vi "Adjust_PID-Controller.vi"() -> ()   [LabVIEW 2018]
uses:
  <vilib>/robotics/Steering/Wheel/Rotation Direction.ctl
  <vilib>/robotics/Steering/Wheel/Wheel Parameters.ctl
  <vilib>/Studica/Studica Toolkit/Background/Mxp Selection.ctl
  <vilib>/robotics/Steering/Omnidirectional Wheel/NI_Robotics_Omnidirectional Wheel.lvclass
  C:/Program Files (x86)/National Instruments/LabVIEW 2018/vi.lib/robotics/Steering/Wheel/NI_Robotics_Wheel.lvclass
  <vilib>/robotics/Steering/Omnidirectional Wheel/Create Omnidirectional Wheel.vi
  <vilib>/robotics/Steering/Steering Frame/Create User Defined Steering Frame.vi
  <vilib>/robotics/Steering/Steering Frame/Apply Steering Frame Velocity to Motors.vi
  <vilib>/robotics/Steering/Wheel/NI_Robotics_Wheel.lvclass
  <vilib>/robotics/Steering/Steering Frame/NI_Robotics_Steering Frame.lvclass
panel:
  in  "PID gains":T1(array[cluster]) {"proportional gain (Kc)" step=0.01; "integral time (Ti, min)" min=0.0 step=0.0001; "derivative time (Td, min)" step=0.0001}
  out "PID-Output":dbl[](array[numeric])
  out "Actual-SpeedList":dbl[](array[numeric])
  out "Desired Velocity":dbl[](array[numeric])=[-0.0, -0.0, -0.0]
  in  "theta":dbl
  in  "y":dbl
  in  "x":dbl
  in  "Reset Encoders":bool
  out "Tick Count(uSec)":u32=1278617 caption="Tick Count(Ticks)"
  in  "Wheel Index Adjustment (2, 0, 1)":i32[](array[numeric])=[2, 0, 1]
  in  "stop":bool
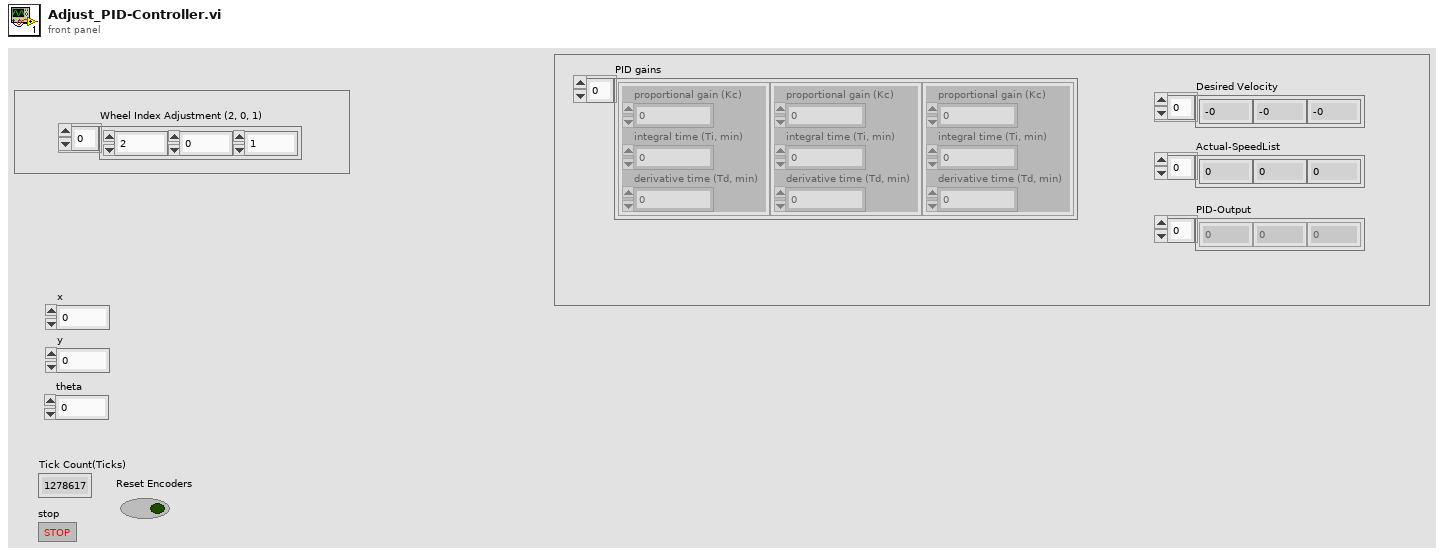
[diagram p1: front panel]
types:
  T1 = cluster{"proportional gain (Kc)":dbl, "integral time (Ti, min)":dbl, "derivative time (Td, min)":dbl}[]
  T2 = typedef "NI_Robotics_Wheel.lvclass/Wheel Parameters.ctl" = cluster{"wheel radius":dbl, "gear ratio":dbl, "forward rotation direction":T3}
  T3 = typedef "NI_Robotics_Wheel.lvclass/Rotation Direction.ctl" = u16
  T4 = typedef "Mxp Selection.ctl" = enum16{"MXP A", "MXP B"}
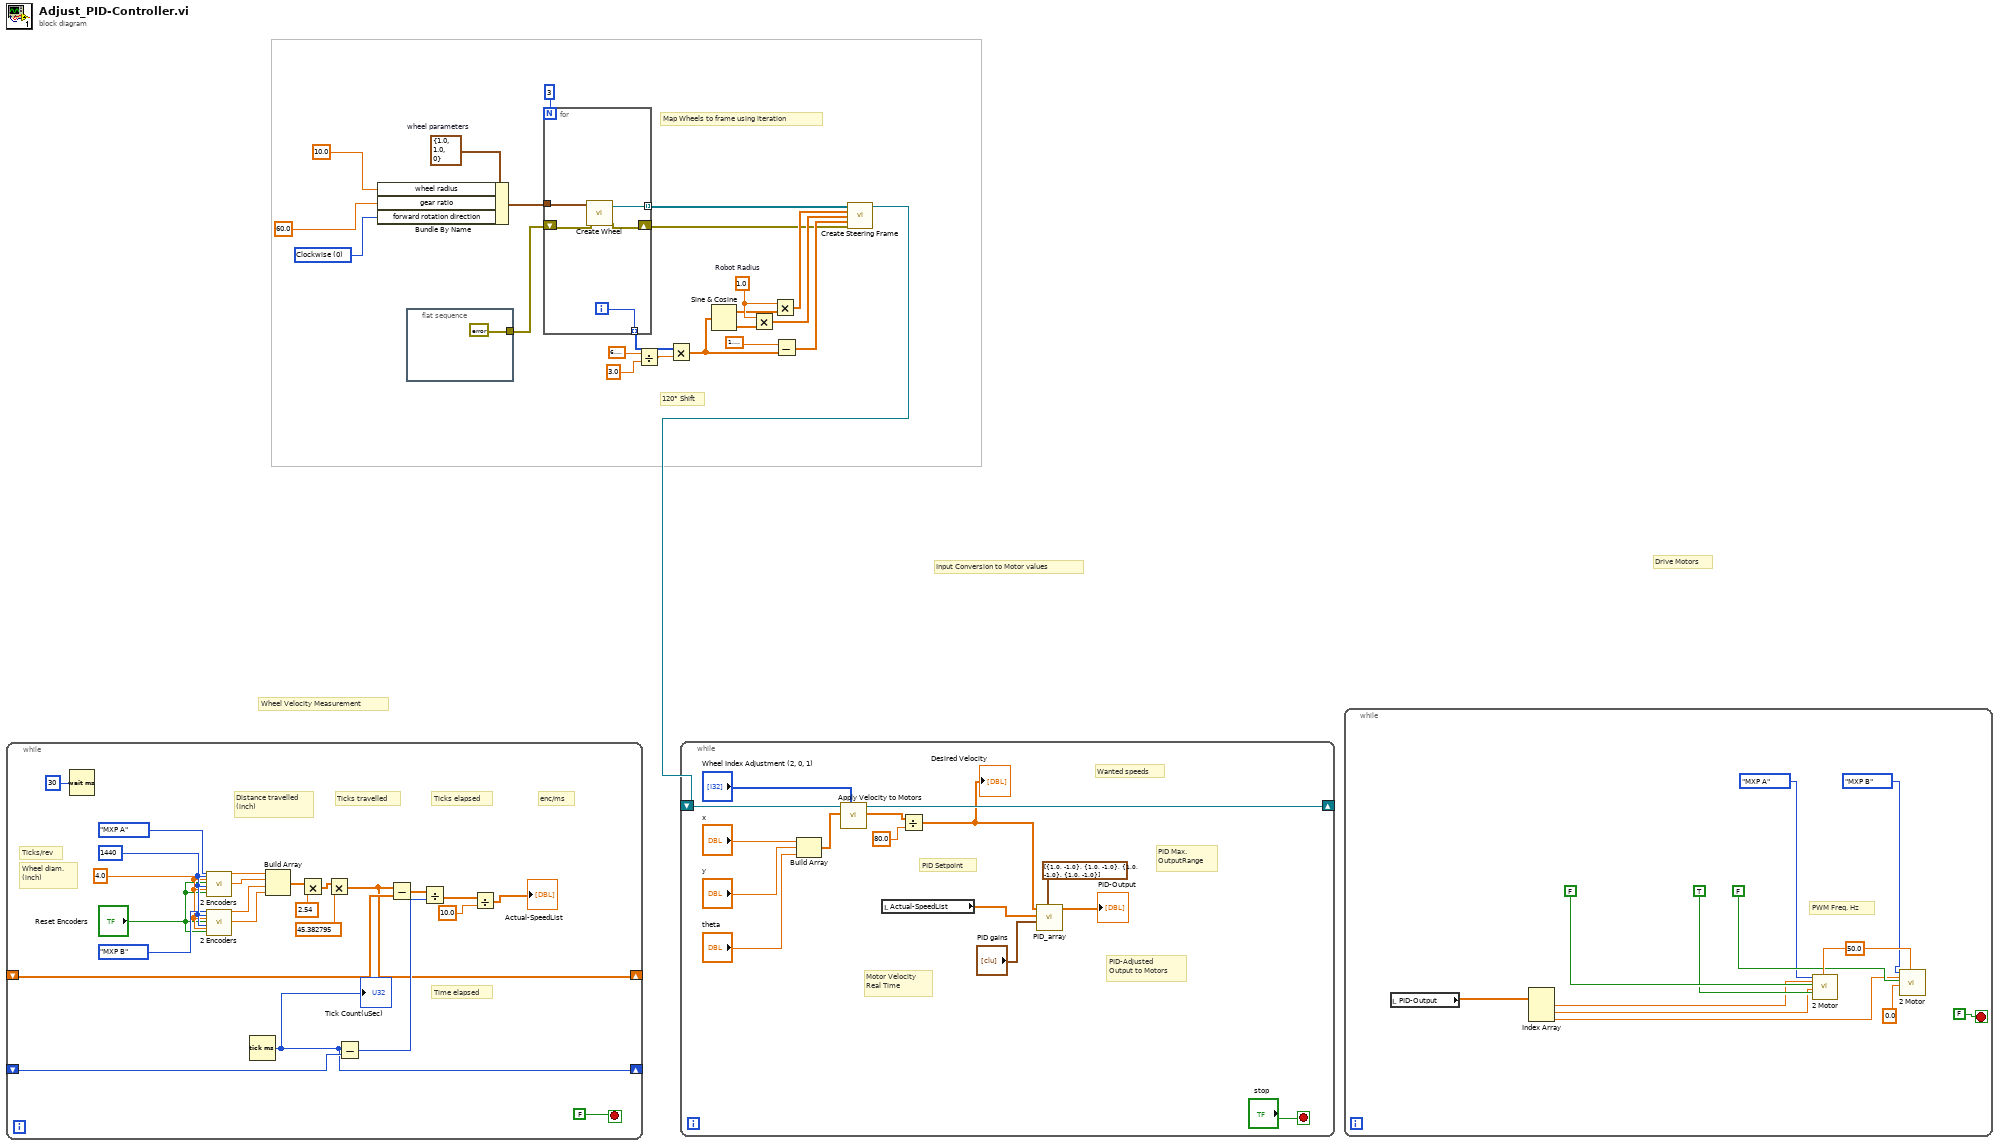
[diagram p0: block diagram]
diagram:
  w22 = T2 {"wheel radius"=1.0, "gear ratio"=1.0, "forward rotation direction"=0}  # wheel parameters
  w8 = T3 0 items=["Clockwise", "Counterclockwise"] ("forward rotation direction")
  w13 = 1.0  # Robot Radius
  # "Drive Motors"
  # "Wheel Velocity Measurement"
  # "120° Shift"
  # "Map Wheels to frame using iteration"
  # "Input Conversion to Motor values"
  n1 = while {
    shift-right: [w29] -> _
    shift-left: _ -> [w34]
    shift-right: [w30] -> _
    shift-left: _ -> [w32]
    stop <- FALSE stop-if-true
    w27 = 4.0 ("Wheel Diameter M1 (inches)")
    w37 = u32 1440 ("Ticks Per Rev M0")
    # "Ticks travelled"
    # "Distance travelled\n(inch)"
    # "Wheel diam.\n(inch)"
    # "Ticks/rev"
    # "Ticks elapsed"
    # "Time elapsed"
    # "enc/ms"
    n2 = Wait (ms)(milliseconds to wait=u32 30) -> ()  [unwired: 1 out]
    n3 = call <vilib>:"2 Encoders.vi"("Mxp Side"=Mxp_Selection."MXP A", "Ticks Per Rev M0"=w37, "Wheel Diameter M0 (inches)"=w27, "Reset Encoder 0"="Reset Encoders", "Ticks Per Rev M1"=w37, "Wheel Diameter M1 (inches)"=w27, "Reset Encoder 1"="Reset Encoders") -> ("Distance M0 (inches)"=w38:dbl, "Distance M1 (inches)"=w39:dbl)  [unwired: 18 in, 1 out]
    n4 = call <vilib>:"2 Encoders.vi"("Mxp Side"=Mxp_Selection."MXP B", "Ticks Per Rev M0"=w37, "Wheel Diameter M0 (inches)"=w27, "Reset Encoder 0"="Reset Encoders", "Ticks Per Rev M1"=w37, "Wheel Diameter M1 (inches)"=w27, "Reset Encoder 1"="Reset Encoders") -> ("Distance M0 (inches)"=w40:dbl, "Distance M1 (inches)"=w28:dbl)  [unwired: 18 in, 1 out]
    n5 = Tick Count (ms)() -> (millisecond timer value=w30:u32)
    "Tick Count(uSec)" <- w30
    n6 = Build Array(w38, w39, w40, w28) -> (w42:dbl[])
    n7 = Multiply(x=w42, y=2.54) -> (x*y=w43:dbl[])
    n8 = Multiply(x=w43, y=45.382795) -> (x*y=w29:dbl[])
    n9 = Subtract(x=w30, y=w32) -> (x-y=w45:u32)
    n10 = Subtract(x=w29, y=w34) -> (x-y=w33:dbl[])
    n11 = Divide(x=w33, y=w45) -> (x/y=w25:dbl[])
    n12 = Divide(x=w25, y=10.0) -> (x/y=→"Actual-SpeedList":dbl[])
  }
  n13 = Bundle By Name(cluster=w22, "wheel radius"=10.0, "gear ratio"=60.0 ("wheel radius"), "forward rotation direction"=w8) -> (w20:T2)
  n14 = flat-sequence {
    tunnel: [errorcluster {"status"=FALSE, "code"=0, "source"=""} ("error out")] -> w19
    frame #0 {
    }
  }
  n15 = for {
    N: 3 -> [_]
    shift-right: [w51] -> w6
    shift-left: w19 -> [w52]
    tunnel: [w50] -> w18 mode=indexing
    tunnel: w20 -> [w49]
    tunnel: [w48] -> w14 mode=indexing
    i -> [w48]
    n16 = call-poly <vilib>:"Create Wheel.vi"("error in (no error)"=w52, "wheel parameters"=w49) -> ("error out"=w51:errorcluster, "omni wheel out"=w50:refnum<class "NI_Robotics_Omnidirectional Wheel.lvclass">)  [unwired: 8 in]
  }
  n17 = Divide(x=6.283185307179586, y=3.0) -> (x/y=w15:dbl)
  n18 = Multiply(x=w14, y=w15) -> (x*y=w3:dbl[])
  n19 = Sine & Cosine(0:w3) -> (1:w5:dbl[], 2:w4:dbl[])
  n20 = Multiply(x=w13, y=w4) -> (x*y=w11:dbl[])
  n21 = Multiply(x=w13, y=w5) -> (x*y=w12:dbl[])
  n22 = Subtract(x=1.5707963267948966, y=w3) -> (x-y=w9:dbl[])
  n23 = call-poly <vilib>:"Create Steering Frame.vi"("wheel frame angles (rad)"=w9, "error in (no error)"=w6, "wheel y positions"=w11, "wheel x positions"=w12, "wheels"=w18) -> ("steering frame out"=w2:refnum<class "NI_Robotics_Steering Frame.lvclass">)  [unwired: 5 in, 1 out]
  n24 = while {
    shift-right: [w65] -> _
    shift-left: w2 -> [w66]
    stop <- "stop" stop-if-true
    # "Wanted speeds"
    # "PID-Adjusted\nOutput to Motors"
    # "Motor Velocity\nReal Time"
    # "PID Max. \nOutputRange"
    # "PID Setpoint"
    n25 = Build Array("x", "y", "theta") -> (w63:dbl[])
    n26 = call-poly <vilib>:"Apply Velocity to Motors.vi"("wheel indexes"="Wheel Index Adjustment (2, 0, 1)", "steering frame velocity"=w63, "steering frame in"=w66) -> ("ccw motor velocity setpoints"=w59:dbl[], "steering frame out"=w65:refnum<class "NI_Robotics_Steering Frame.lvclass">)  [unwired: 4 in, 3 out]
    n27 = local read "Actual-SpeedList"() -> (w56:dbl[])
    n28 = Divide(x=w59, y=80.0 ("Wheel Diameter M1 (inches)")) -> (x/y=w57:dbl[])
    "Desired Velocity" <- w57
    n29 = call "PID_array.vi"("output range"=cluster{"output high":dbl, "output low":dbl}[] [{"output high"=1.0, "output low"=-1.0}, {"output high"=1.0, "output low"=-1.0}, {"output high"=1.0, "output low"=-1.0}, {"output high"=1.0, "output low"=-1.0}], "PID gains"="PID gains", "process variable"=w56, "setpoint"=w57) -> ("output"=→"PID-Output":dbl[])  [unwired: 6 in, 1 out]
  }
  n30 = while {
    stop <- FALSE stop-if-true
    w78 = 50.0 ("Frequency [Hz]")
    # "PWM Freq. Hz"
    n31 = local read "PID-Output"() -> (w79:dbl[])
    n32 = Index Array(array=w79) -> (element #1=w74:dbl, element #2=w68:dbl, element #3=w73:dbl)  [unwired: 3 in]
    n33 = call <vilib>:"2 Motor.vi"("Mxp Side"=Mxp_Selection."MXP A", "Speed M0"=w74, "Invert M0"=FALSE, "Speed M1"=w68, "Invert M1"=TRUE ("Invert M0"), "Frequency [Hz]"=w78) -> ()  [unwired: 13 in, 1 out]
    n34 = call <vilib>:"2 Motor.vi"("Mxp Side"=Mxp_Selection."MXP B", "Speed M0"=w73, "Invert M0"=FALSE, "Speed M1"=0.0, "Frequency [Hz]"=w78) -> ()  [unwired: 14 in, 1 out]
  }
